vi "Drive Loop Initialize.vi"(11 "name (unnamed)":string) -> (2 "Numeric":u32, 3 "Drive Loop Cluster":T1)   [LabVIEW 2015]
uses:
  Drive Code Support/Drive Code Bundle.ctl
  Drive Code Support/Sensor Cluster.ctl
  Drive Code Support/Camera Cluster.ctl
  Drive Code Support/Drive Code Notifier.ctl
  Drive Code Support/Drive Code Command.ctl
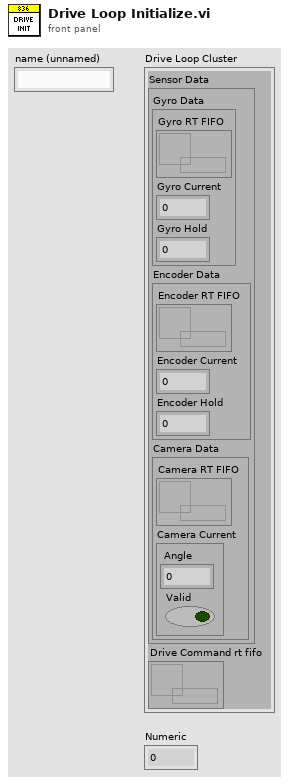
[diagram p1: front panel]
types:
  T1 = typedef "Drive Code Bundle.ctl" = cluster{"Sensor Data":T2, "Drive Command rt fifo":refnum<k33>}
  T2 = typedef "Sensor Cluster.ctl" = cluster{"Gyro Data":cluster{"Gyro RT FIFO":refnum<k33>, "Gyro Current":dbl, "Gyro Hold":dbl}, "Encoder Data":cluster{"Encoder RT FIFO":refnum<k33>, "Encoder Current":dbl, "Encoder Hold":dbl}, "Camera Data":cluster{"Camera RT FIFO":refnum<k33>, "Camera Current":T3}}
  T3 = typedef "Camera Cluster.ctl" = cluster{" Angle":dbl, "Valid":bool}
  T4 = typedef "Drive Code Notifier.ctl" = cluster{"Command":T5, "Parameter A":dbl, "Parameter B":dbl, "Parameter C":dbl, "Absolute?":bool}
  T5 = typedef "Drive Code Command.ctl" = enum16{"Do Nothing", "Manual", "Drive Continuous", "Turn", "Drive Distance", "Hold Position", "Hold Yaw", "Follow Camera", "Turn to Camera"}
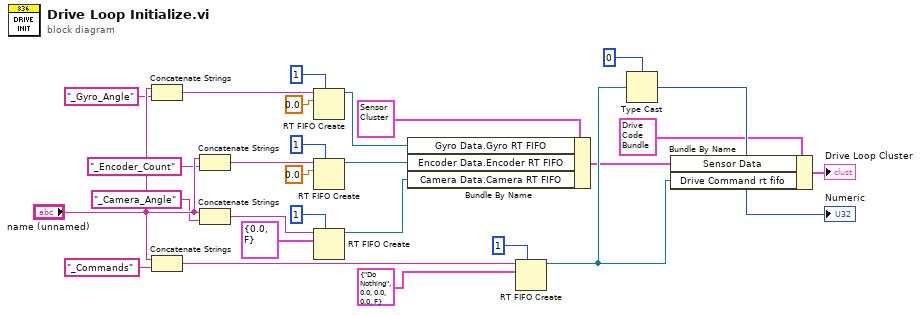
[diagram p0: block diagram]
diagram:
  n1 = Concatenate Strings("name (unnamed)", "_Gyro_Angle" ("string")) -> (w12:string)
  n2 = Concatenate Strings("name (unnamed)", "_Commands" ("string")) -> (w2:string)
  n3 = Concatenate Strings("name (unnamed)", "_Encoder_Count" ("string")) -> (w11:string)
  n4 = Concatenate Strings("name (unnamed)", "_Camera_Angle" ("string")) -> (w8:string)
  n5 = RT FIFO Create(0:w12, 1:0.0, 4:u32 1 ("size (10)")) -> (8:w18:refnum<k33>)  [unwired: 5 in, 2 out]
  n6 = RT FIFO Create(0:w11, 1:0.0, 4:u32 1 ("size (10)")) -> (8:w19:refnum<k33>)  [unwired: 5 in, 2 out]
  n7 = RT FIFO Create(0:w8, 1:T3 {" Angle"=0.0, "Valid"=FALSE}, 4:u32 1 ("size (10)")) -> (8:w20:refnum<k33>)  [unwired: 5 in, 2 out]
  n8 = Bundle By Name(cluster=T2 {"Gyro Data"={"Gyro RT FIFO"=refnum, "Gyro Current"=0.0, "Gyro Hold"=0.0}, "Encoder Data"={"Encoder RT FIFO"=refnum, "Encoder Current"=0.0, "Encoder Hold"=0.0}, "Camera Data"={"Camera RT FIFO"=refnum, "Camera Current"={" Angle"=0.0, "Valid"=FALSE}}}, "Gyro Data.Gyro RT FIFO"=w18, "Encoder Data.Encoder RT FIFO"=w19, "Camera Data.Camera RT FIFO"=w20) -> (w22:T2)
  n9 = RT FIFO Create(0:w2, 1:T4 {"Command"=enum."Do Nothing", "Parameter A"=0.0, "Parameter B"=0.0, "Parameter C"=0.0, "Absolute?"=FALSE}, 4:u32 1 ("size (10)")) -> (8:w26:refnum<k33>)  [unwired: 5 in, 2 out]
  n10 = Type Cast(type=u32 0, x=w26) -> (*(type *) &x=→"Numeric":u32)
  n11 = Bundle By Name(cluster=T1 {"Sensor Data"={"Gyro Data"={"Gyro RT FIFO"=refnum, "Gyro Current"=0.0, "Gyro Hold"=0.0}, "Encoder Data"={"Encoder RT FIFO"=refnum, "Encoder Current"=0.0, "Encoder Hold"=0.0}, "Camera Data"={"Camera RT FIFO"=refnum, "Camera Current"={" Angle"=0.0, "Valid"=FALSE}}}, "Drive Command rt fifo"=refnum} ("Cluster"), "Sensor Data"=w22, "Drive Command rt fifo"=w26) -> (→"Drive Loop Cluster":T1)
